vi "Kepco cfg load list.vi"(8 "error in (no error)":errorcluster {"code" format="%.0x"}, 9 "Simulation":T1, 10 "Channel parsed command info":T2, 11 "input cluster":refnum<class "KepcoBOP.lvclass">) -> (0 "error out":errorcluster, 2 "new commands":string, 3 "output cluster":refnum<class "KepcoBOP.lvclass">)   [LabVIEW 2020, in "KepcoBOP.lvclass"]
uses:
  KepcoBOP.lvclass
  Shared/Device Driver/channel parsed cmd cluster.ctl
  shared/OnOffTypeDef.ctl
  KepcoBOP.lvclass/KepcoBOP.ctl
  shared/CompressAndUpdate(Poly)/CompressAndUpdate(Enum).vi
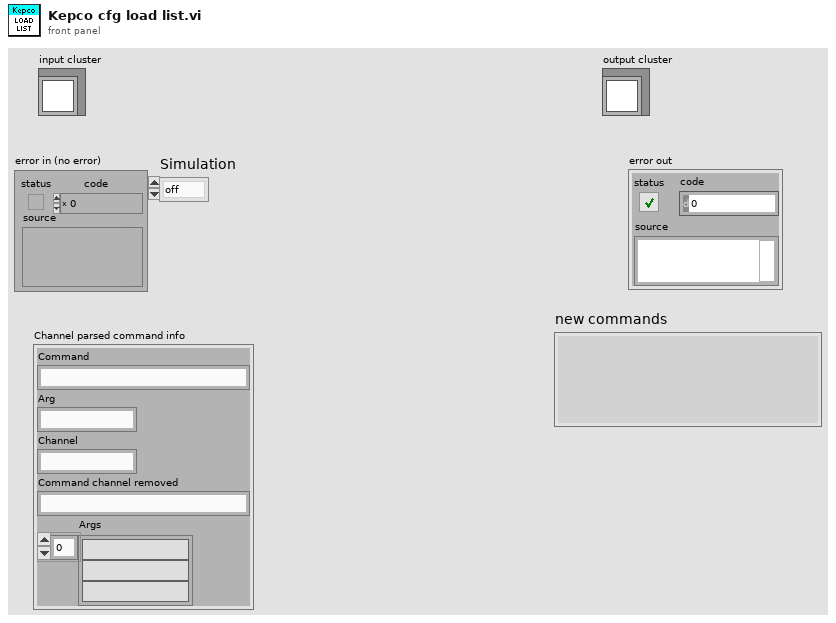
[diagram p1: front panel]
types:
  T1 = typedef "OnOffTypeDef.ctl" = enum16{"off", "on"}
  T2 = typedef "channel parsed cmd cluster.ctl" = cluster{"Command":string, "Arg":string, "Channel":string, "Command channel removed":string, "Args":string[]}
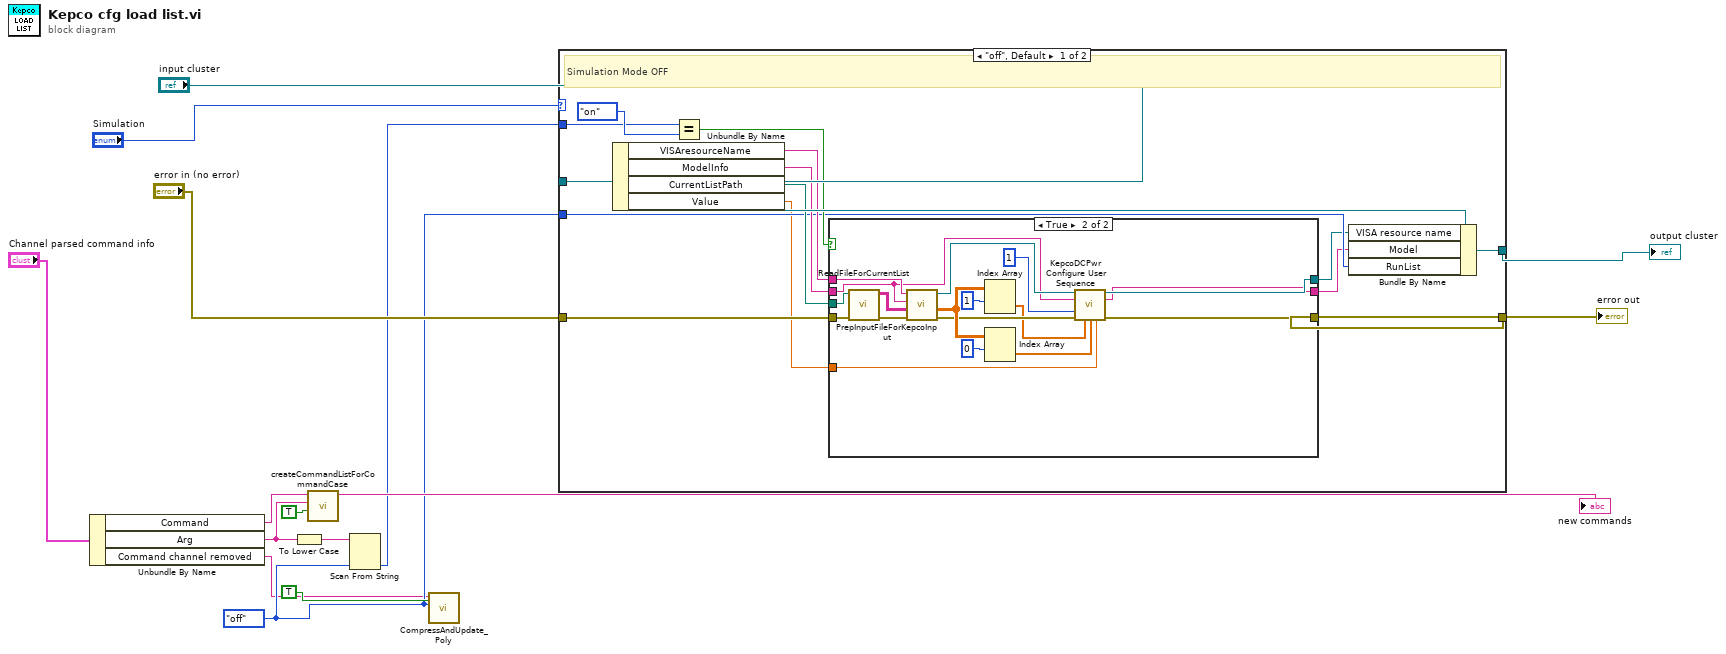
[diagram p0: block diagram]
diagram:
  w2 = enum16{"off", "on"}."off"
  n1 = Unbundle By Name("Channel parsed command info") -> ("Command"=w14:string, "Arg"=w4:string, "Command channel removed"=w1:string)
  n2 = To Lower Case(string=w4) -> (all lower case string=w5:string)
  n3 = call "createCommandListForCommandCase.vi"("immediate Check (only once)"=TRUE, "setvalue"=w4, "command"=w14) -> ("new commands"=→"new commands":string)  [unwired: 8 in]
  n4 = Scan From String(input string=w5, default 1=w2) -> (output 1=w3:enum16{"off", "on"})  [unwired: 3 in, 3 out]
  n5 = call-poly "CompressAndUpdate_Poly.vi"("force CVT update (false)"=TRUE ("force CVT update"), "enum variant"=w2, "command or variable name"=w1) -> ()  [unwired: 8 in, 1 out]
  n6 = case shown="\"off\", Default" "Simulation" {
    tunnel: [w23 w51] -> w9
    tunnel: "input cluster" -> [w29 w52]
    tunnel: "error in (no error)" -> [w24 w51]
    tunnel: [w28 w52] -> w10
    tunnel: w3 -> [w26 _]
    tunnel: w2 -> [w19 _]
    frame "off", Default {
      # "Simulation Mode OFF"
      n7 = Unbundle By Name(w29) -> ("VISAresourceName"=w22:string, "ModelInfo"=w21:string, "CurrentListPath"=w20:path, "Value"=w16:dbl)
      n8 = Equal?(x=w26, y=enum16{"off", "on"}."on") -> (x = y?=w25:bool)
      n9 = case shown="True" w25 {
        tunnel: w24 -> [w31 w50]
        tunnel: w22 -> [w30 w47]
        tunnel: w21 -> [w32 w41]
        tunnel: [w32 w35] -> w17
        tunnel: [w31 w34] -> w23
        tunnel: w20 -> [_ w46]
        tunnel: [w30 w36] -> w18
        tunnel: w16 -> [_ w33]
        frame False {
        }
        frame True {
          n10 = call "ReadFileForCurrentList.vi"("error in"=w50, "CurrentList file path"=w46) -> ("error out"=w48:errorcluster, "CurrentList out"=w49:string[][])  [unwired: 8 in]
          n11 = call "PrepInputFileForKepcoInput.vi"("error in"=w48, "Waveform List In"=w49, "Model In"=w41, "VISA Session In"=w47) -> ("error out"=w39:errorcluster, "CurrentList"=w43:dbl[][], "VISA Session Out"=w42:refnum<visa-resource-name>)  [unwired: 4 in, 1 out]
          n12 = Index Array(array=w43, index (row)=1 ("index")) -> (element=w38:dbl[])  [unwired: 1 in]
          n13 = Index Array(array=w43, index (row)=0 ("index")) -> (element=w37:dbl[])  [unwired: 1 in]
          n14 = call "KepcoDCPwr Configure User Sequence.vi"("VISA Session"=w42, "Model In"=w41, "# of Cycles"=1, "error in (no error)"=w39, "Dwell (sec)"=w38, "List Data"=w37, "Limit Value"=w33) -> ("VISA Session Out"=w36:refnum<visa-resource-name>, "Model Out"=w35:string, "error out"=w34:errorcluster)  [unwired: 1 in, 5 out]
        }
      }
      n15 = Bundle By Name(cluster=w29, "VISA resource name"=w18, "Model"=w17, "RunList"=w19) -> (w28:refnum<class "KepcoBOP.lvclass">)
    }
    frame "on" {
      # "Simulation Mode ON"
    }
  }
  "output cluster" <- w10
  "error out" <- w9
